vi "Close Ref.vi"(8 "error in (no error)":errorcluster, 11 "PXIe 2737 in":refnum<class "PXIe 2737.lvclass">) -> (0 "error out":errorcluster, 3 "PXIe 2737 out":refnum<class "PXIe 2737.lvclass">)   [LabVIEW 2023, in "S-Matrix.lvlib" / "PXIe 2737.lvclass"]
uses:
  PXIe 2737.lvclass
  PXIe 2737.lvclass/PXIe 2737.ctl
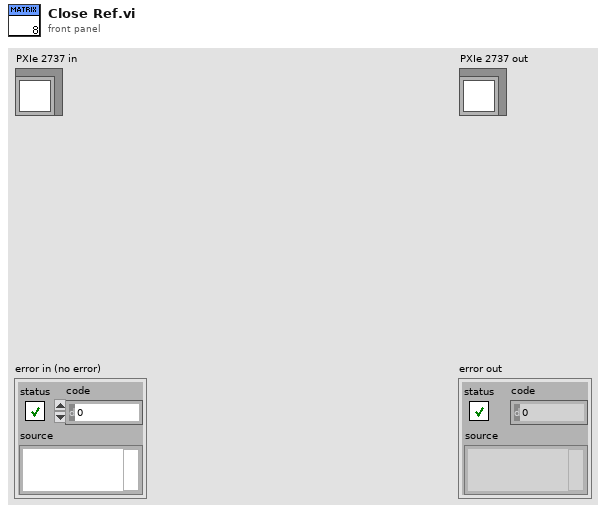
[diagram p1: front panel]
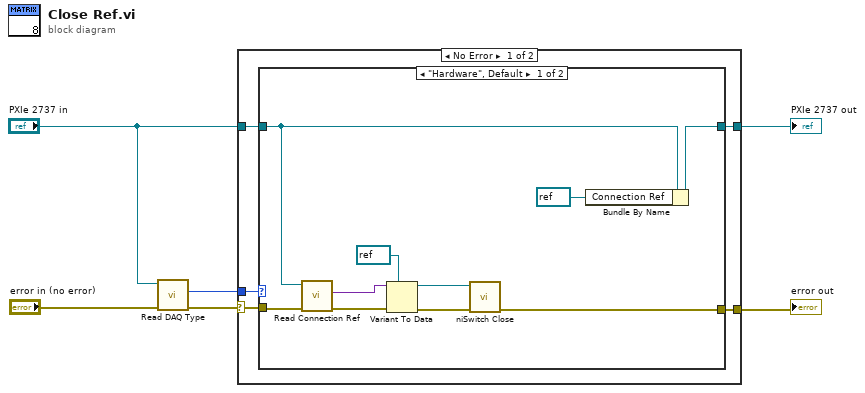
[diagram p0: block diagram]
diagram:
  n1 = call-dynamic "Read DAQ Type.vi"("error in (no error)"="error in (no error)", "PXIe 2737 in"="PXIe 2737 in") -> ("error out"=w5:errorcluster, "DAQ Type"=w4:enum16{"Hardware", "Simulation"})  [unwired: 7 in, 1 out]
  n2 = case shown="No Error" w5 {
    selector: w5 -> [w11 w24]
    tunnel: w4 -> [w10 _]
    tunnel: "PXIe 2737 in" -> [w9 w25]
    tunnel: [w8 w25] -> w2
    tunnel: [w7 w24] -> w1
    frame No Error {
      n3 = case shown="\"Hardware\", Default" w10 {
        tunnel: w11 -> [w21 w22]
        tunnel: w9 -> [w15 w23]
        tunnel: [w13 w23] -> w8
        tunnel: [w14 w22] -> w7
        frame "Hardware", Default {
          n4 = call-dynamic "Read Connection Ref.vi"("error in (no error)"=w21, "PXIe 2737 in"=w15) -> ("error out"=w20:errorcluster, "Connection Ref"=w19:variant)  [unwired: 7 in, 1 out]
          n5 = Variant To Data(error in=w20, type=refnum<k15> refnum ("instrument handle"), Variant=w19) -> (data=w17:refnum<k15>, error out=w16:errorcluster)
          n6 = call <instrlib>:"niSwitch Close.vi"("error in (no error)"=w16, "instrument handle"=w17) -> ("error out"=w14:errorcluster)  [unwired: 9 in]
          n7 = Bundle By Name(cluster=w15, "Connection Ref"=refnum<k15> refnum ("instrument handle")) -> (w13:refnum<class "PXIe 2737.lvclass">)
        }
        frame "Simulation" {
        }
      }
    }
    frame Error {
    }
  }
  "error out" <- w1
  "PXIe 2737 out" <- w2
